vi "test JSON id.vi"(8 "error in (no error)":errorcluster, 11 "TestCase in":refnum<class "JSONAble Tests.lvclass">) -> (0 "error out":errorcluster, 3 "TestCase out":refnum<class "JSONAble Tests.lvclass">)   [LabVIEW 2017, in "JSONAble Tests.lvclass"]
uses:
  JSONAble Tests.lvclass
  Classes/id/id.lvclass
  <vilib>/addons/_JKI Toolkits/VI Tester/TestCase.llb/TestCase.lvclass
  <vilib>/National Instruments/Variant JSON API/Variant JSON API.lvlib
  C:/Program Files (x86)/National Instruments/LabVIEW 2017/vi.lib/addons/_JKI Toolkits/VI Tester/TestCase.llb/TestCase.lvclass
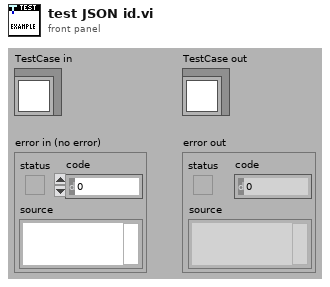
[diagram p1: front panel]
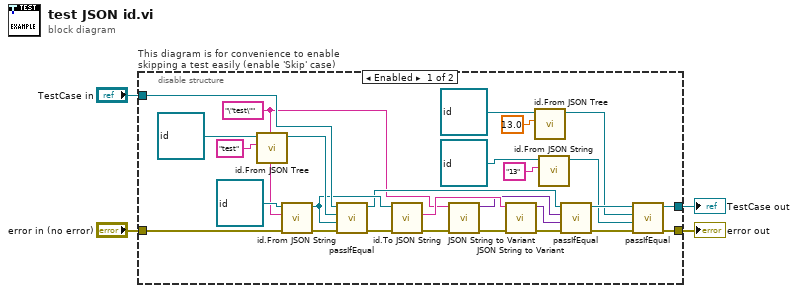
[diagram p0: block diagram]
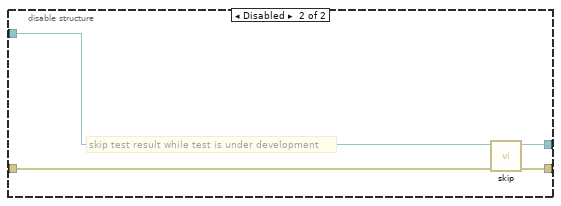
[diagram p2: hidden frame]
diagram:
  n1 = disable-structure "This diagram is for convenience to enable skipping a test easily (enable 'Skip' case)" shown="Enabled" {
    disable-tunnel: "TestCase in" -> [w29 w35]
    disable-tunnel: [w11 w33] -> w1
    disable-tunnel: [w13 w34] -> w3
    disable-tunnel: "error in (no error)" -> [w27 w32]
    frame Enabled {
      w20 = "\"test\"" ("JSON String")
      n2 = call "id.From JSON Tree.vi"("JSON Value in"="test", "id in"=refnum<class "id.lvclass"> refnum ("id.lvclass")) -> ("id out"=w28:refnum<class "id.lvclass">)  [unwired: 8 in, 1 out]
      n3 = call "id.From JSON String.vi"("error in (no error)"=w27, "JSON String"=w20, "id in"=refnum<class "id.lvclass"> refnum ("id.lvclass")) -> ("error out"=w25:errorcluster, "id out"=w26:refnum<class "id.lvclass">)  [unwired: 7 in]
      n4 = call-dynamic "passIfEqual.vi"("error in (no error)"=w25, "y"=w26, "x"=w28, "TestCase in"=w29) -> ("error out"=w24:errorcluster, "TestCase out"=w22:refnum<class "JSONAble Tests.lvclass">)  [unwired: 6 in]
      n5 = call "id.To JSON String.vi"("error in (no error)"=w24, "id in"=w26) -> ("error out"=w17:errorcluster, "JSON String"=w21:string)  [unwired: 7 in, 1 out]
      n6 = call <vilib>:"JSON String to Variant.vi"("error in (no error)"=w17, "JSON String"=w20) -> ("error out"=w16:errorcluster, "Variant out"=w18:variant)  [unwired: 8 in]
      n7 = call <vilib>:"JSON String to Variant.vi"("error in (no error)"=w16, "JSON String"=w21) -> ("error out"=w15:errorcluster, "Variant out"=w19:variant)  [unwired: 8 in]
      n8 = call "id.From JSON Tree.vi"("JSON Value in"=13.0, "id in"=refnum<class "id.lvclass"> refnum ("id.lvclass")) -> ("id out"=w7:refnum<class "id.lvclass">)  [unwired: 8 in, 1 out]
      n9 = call "id.From JSON String.vi"("JSON String"="13", "id in"=refnum<class "id.lvclass"> refnum ("id.lvclass")) -> ("id out"=w6:refnum<class "id.lvclass">)  [unwired: 8 in, 1 out]
      n10 = call-dynamic "passIfEqual.vi"("error in (no error)"=w15, "y"=w19, "x"=w18, "TestCase in"=w22) -> ("error out"=w23:errorcluster, "TestCase out"=w12:refnum<class "JSONAble Tests.lvclass">)  [unwired: 6 in]
      n11 = call-dynamic "passIfEqual.vi"("error in (no error)"=w23, "y"=w6, "x"=w7, "TestCase in"=w12) -> ("error out"=w13:errorcluster, "TestCase out"=w11:refnum<class "JSONAble Tests.lvclass">)  [unwired: 6 in]
    }
    frame Disabled {
      # "skip test result while test is under development"
      n12 = call <vilib>:"skip.vi"("error in (no error)"=w32, "TestCase in"=w35) -> ("error out"=w34:errorcluster, "TestCase out"=w33:refnum<class "JSONAble Tests.lvclass">)  [unwired: 8 in]
    }
  }
  "error out" <- w3
  "TestCase out" <- w1
